vi "Data_folder_Path.vi"(1 "seconds":dbl, 2 "ProjectNumberIn":string, 3 "SetProjectNumber":bool, 4 "FlushHierarchy":bool, 5 "Data Type":string) -> (0 "Data Folder":path)   [LabVIEW 2011]
uses:
  Globals/Constants_global.vi
  Globals/Preference_global.vi
panel:
  out "ProjectNo":string
  out "Hierarchy":string[](array[string])
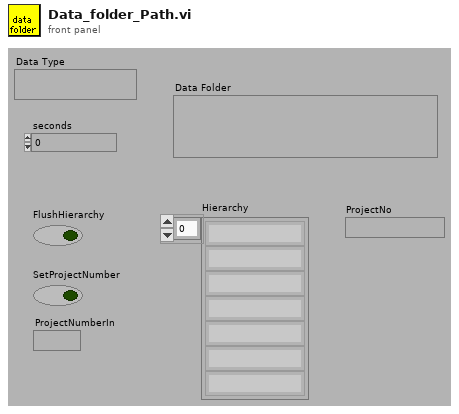
[diagram p1: front panel]
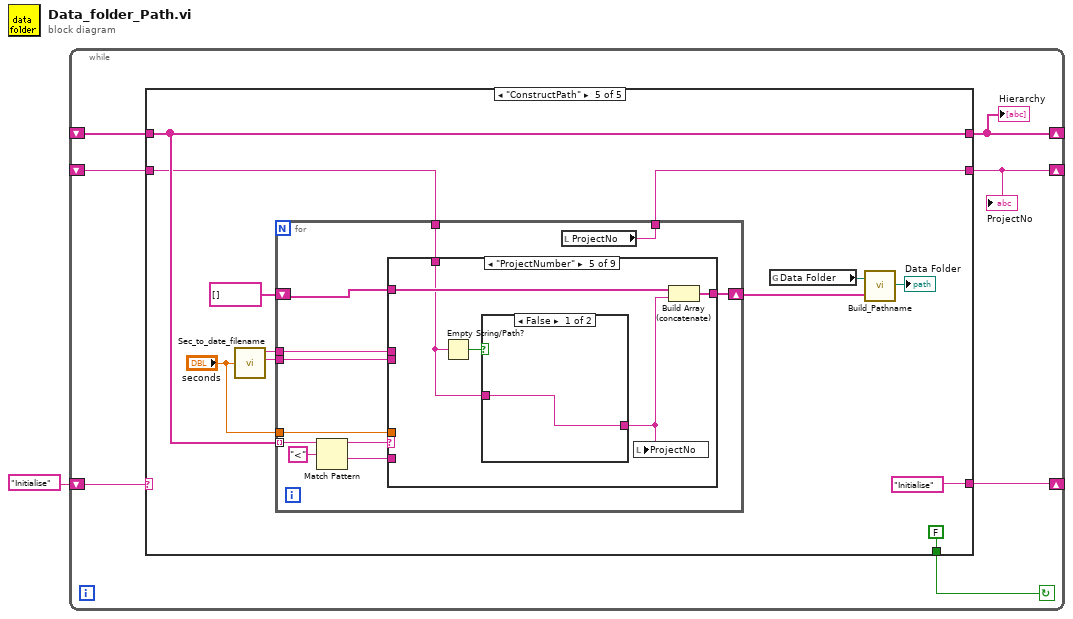
[diagram p0: block diagram]
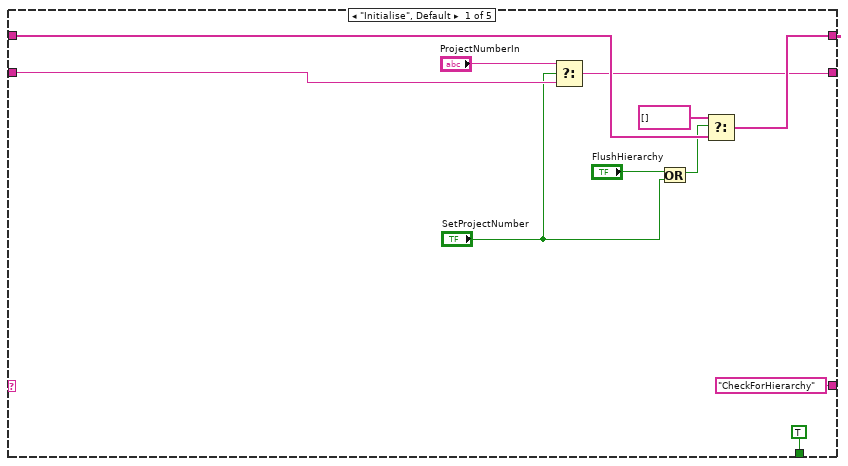
[diagram p2: hidden frame]
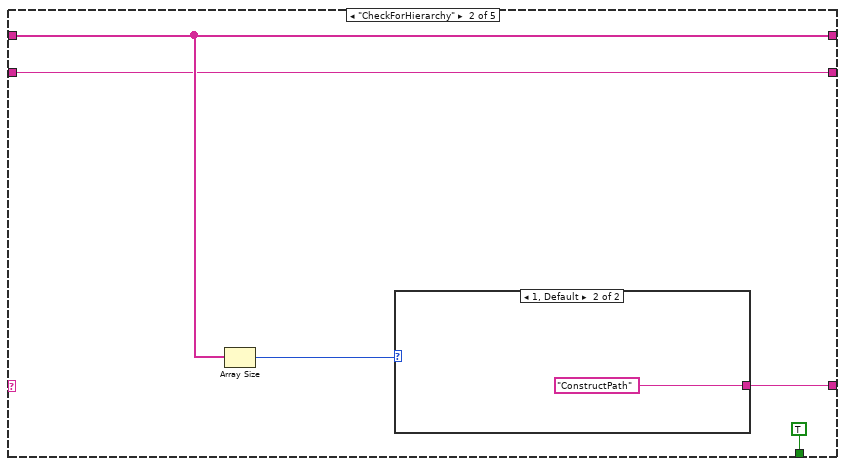
[diagram p3: hidden frame]
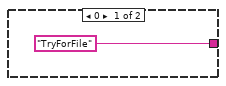
[diagram p4: hidden frame]
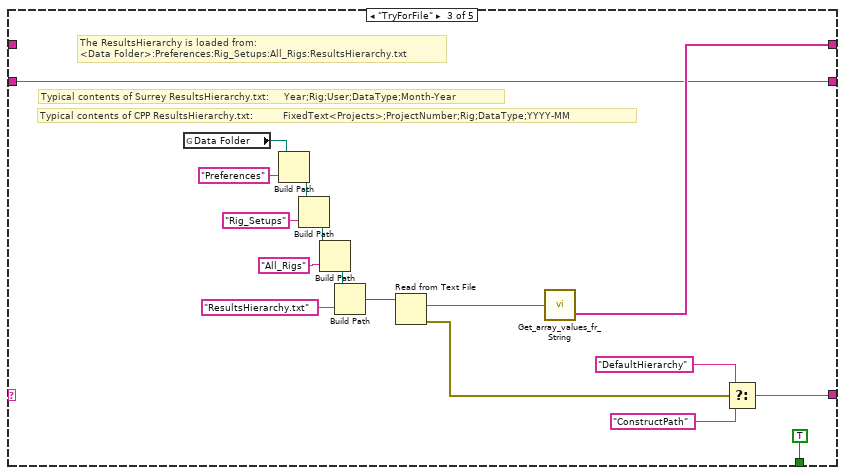
[diagram p5: hidden frame]
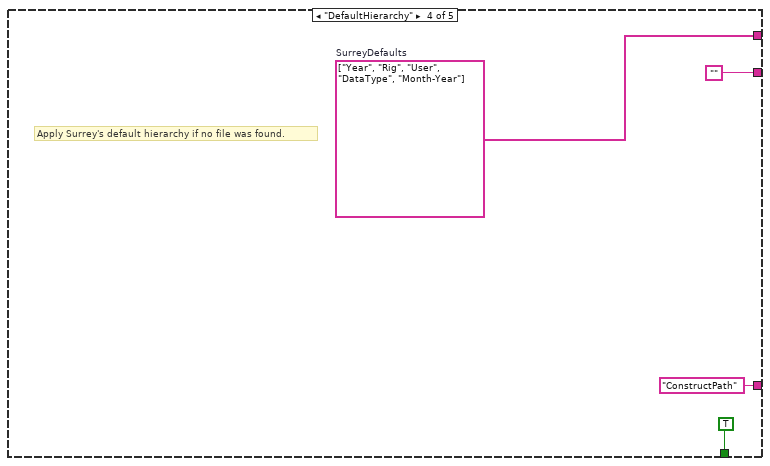
[diagram p6: hidden frame]
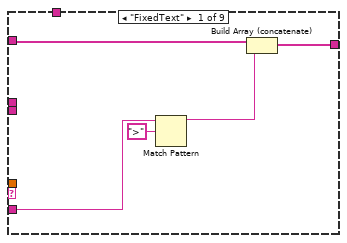
[diagram p7: hidden frame]
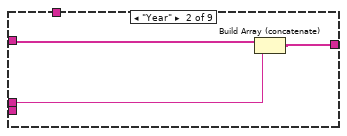
[diagram p8: hidden frame]
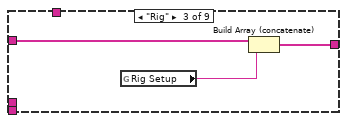
[diagram p9: hidden frame]
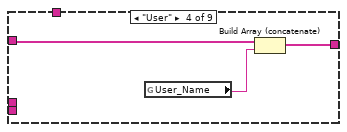
[diagram p10: hidden frame]
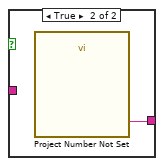
[diagram p11: hidden frame]
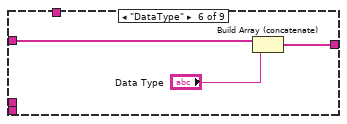
[diagram p12: hidden frame]
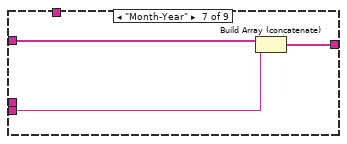
[diagram p13: hidden frame]
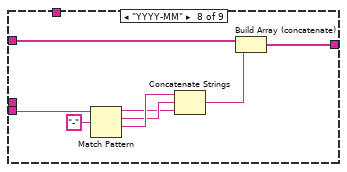
[diagram p14: hidden frame]
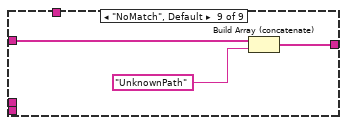
[diagram p15: hidden frame]
diagram:
  n1 = while {
    shift-right: [w6] -> _
    shift-left: _ -> [w7]
    shift-right: [w5] -> _
    shift-left: "Initialise" ("t") -> [w8]
    shift-right: [w3] -> _
    shift-left: _ -> [w4]
    stop <- w2 continue-if-true
    n2 = case shown="\"ConstructPath\"" w8 {
      tunnel: w7 -> [w19 w22 _ _ w52]
      tunnel: [w18 w22 w43 w47 w52] -> w6
      tunnel: ["CheckForHierarchy" ("t") w23 w38 "ConstructPath" ("t") "Initialise" ("t")] -> w5
      tunnel: w4 -> [w14 w21 w35 _ w49]
      tunnel: [w15 w21 w35 "" ("t") w48] -> w3
      tunnel: [TRUE TRUE TRUE TRUE FALSE] -> w2
      frame "Initialise", Default {
        n3 = Select(t="ProjectNumberIn", s="SetProjectNumber", f=w14) -> (s? t:f=w15:string)
        n4 = Or(x="FlushHierarchy", y="SetProjectNumber") -> (x .or. y?=w11:bool)
        n5 = Select(t=string[] [], s=w11, f=w19) -> (s? t:f=w18:string[])
      }
      frame "CheckForHierarchy" {
        n6 = Array Size(array=w22) -> (size(s)=w24:i32)
        n7 = case shown="1, Default" w24 {
          tunnel: ["TryForFile" ("t") "ConstructPath" ("t")] -> w23
          frame 0 {
          }
          frame 1, Default {
          }
        }
      }
      frame "TryForFile" {
        # "The ResultsHierarchy is loaded from:\n<Data Folder>:Preferences:Rig_Setups:All_Rigs:ResultsHierarchy.txt"
        # "Typical contents of CPP ResultsHierarchy.txt:          FixedText<Projects>;ProjectNumber;Rig;DataType;YYYY-MM"
        # "Typical contents of Surrey ResultsHierarchy.txt:     Year;Rig;User;DataType;Month-Year"
        n8 = global read "Constants_global.vi" "Data Folder"() -> (w33:path)
        n9 = Build Path(base path=w33, name or relative path="Preferences") -> (appended path=w29:path)
        n10 = Build Path(base path=w29, name or relative path="Rig_Setups") -> (appended path=w28:path)
        n11 = Build Path(base path=w28, name or relative path="All_Rigs") -> (appended path=w40:path)
        n12 = Build Path(base path=w40, name or relative path="ResultsHierarchy.txt") -> (appended path=w32:path)
        n13 = Read from Text File(file (use dialog)=w32) -> (text=w31:string, error out=w30:errorcluster)  [unwired: 3 in, 2 out]
        n14 = call "Get_array_values_fr_String.vi"("String Value"=w31) -> ("String array"=w43:string[])  [unwired: 1 out]
        n15 = Select(t="DefaultHierarchy", s=w30, f="ConstructPath" ("t")) -> (s? t:f=w38:string)
      }
      frame "DefaultHierarchy" {
        w47 = string[] ["Year", "Rig", "User", "DataType", "Month-Year"]  # SurreyDefaults
        # "Apply Surrey's default hierarchy if no file was found."
      }
      frame "ConstructPath" {
        n16 = call "Sec_to_date_filename.vi"("seconds"="seconds") -> ("Year"=w57:string, "Month"=w56:string)  [unwired: 2 out]
        n17 = for {
          shift-right: [w70] -> w55
          shift-left: string[] [] -> [w69]
          tunnel: w52 -> [w65] mode=indexing
          tunnel: w56 -> [w68]
          tunnel: w57 -> [w67]
          tunnel: "seconds" -> [w66]
          tunnel: w49 -> [w61]
          tunnel: [w60] -> w48
          n18 = Match Pattern(string=w65, regular expression="<") -> (before substring=w64:string, after substring=w62:string)  [unwired: 1 in, 2 out]
          n19 = case shown="\"ProjectNumber\"" w64 {
            tunnel: [w75 w78 w80 w84 w89 w94 w97 w103 w108] -> w70
            tunnel: w69 -> [w74 w77 w79 w82 w88 w93 w96 w102 w107]
            tunnel: w68 -> [_ _ _ _ _ _ w95 w105 _]
            tunnel: w67 -> [_ w76 _ _ _ _ _ _ _]
            tunnel: w66 -> [_ _ _ _ _ _ _ _ _]
            tunnel: w62 -> [w73 _ _ _ _ _ _ _ _]
            tunnel: w61 -> [_ _ _ _ w86 _ _ _ _]
            frame "FixedText" {
              n20 = Match Pattern(string=w73, regular expression=">") -> (before substring=w71:string)  [unwired: 1 in, 3 out]
              n21 = Build Array (concatenate)(w74, w71) -> (w75:string[])
            }
            frame "Year" {
              n22 = Build Array (concatenate)(w77, w76) -> (w78:string[])
            }
            frame "Rig" {
              n23 = global read "Preference_global.vi" "Rig Setup"() -> (w81:string)
              n24 = Build Array (concatenate)(w79, w81) -> (w80:string[])
            }
            frame "User" {
              n25 = global read "Preference_global.vi" "User_Name"() -> (w83:string)
              n26 = Build Array (concatenate)(w82, w83) -> (w84:string[])
            }
            frame "ProjectNumber" {
              n27 = Empty String/Path?(string/path=w86) -> (empty?=w87:bool)
              n28 = case shown="False" w87 {
                tunnel: [w90 w91] -> w85
                tunnel: w86 -> [w90 _]
                frame False {
                }
                frame True {
                  n29 = call "Project Number Not Set"() -> ("ProjectNumber"=w91:string)  [unwired: 17 in, 2 out]
                }
              }
              n30 = local write "ProjectNo"(w85) -> ()
              n31 = Build Array (concatenate)(w88, w85) -> (w89:string[])
            }
            frame "DataType" {
              n32 = Build Array (concatenate)(w93, "Data Type") -> (w94:string[])
            }
            frame "Month-Year" {
              n33 = Build Array (concatenate)(w96, w95) -> (w97:string[])
            }
            frame "YYYY-MM" {
              n34 = Match Pattern(string=w105, regular expression="-") -> (before substring=w99:string, match substring=w100:string, after substring=w101:string)  [unwired: 1 in, 1 out]
              n35 = Concatenate Strings(w101, w100, w99) -> (w98:string)
              n36 = Build Array (concatenate)(w102, w98) -> (w103:string[])
            }
            frame "NoMatch", Default {
              n37 = Build Array (concatenate)(w107, "UnknownPath" ("element")) -> (w108:string[])
            }
          }
          n38 = local read "ProjectNo"() -> (w60:string)
        }
        n39 = global read "Constants_global.vi" "Data Folder"() -> (w53:path)
        n40 = call "Build_Pathname.vi"("Output Array"=w55, "Pathname"=w53) -> ("Appended path"=→"Data Folder":path)
      }
    }
    "Hierarchy" <- w6
    "ProjectNo" <- w3
  }
